vi "诊断标定3 - 副本.vi"(8 "CAN端口":u16(ring), 9 "设备索引号":u16(ring), 10 "CAN卡类型":u32(ring)=21) -> ()   [LabVIEW 2013] (continued)
                n2268 = local read "设备索引号"() -> (w2798:u16)
                n2269 = local read "CAN卡类型"() -> (w2799:u32)
                n2270 = local read "CAN端口"() -> (w2797:u16)
                n2271 = Boolean To (0,1)(Boolean=w2794) -> (0, 1=w2791:i16)
                n2272 = Quotient & Remainder(x=w2788, y=w2789) -> (x-y*floor(x/y)=w2785:dbl)  [unwired: 1 out]
                n2273 = Build Array(i16 1 ("元素"), w2791, w2785, w2784, w2783, w2782, 0.0 ("元素")) -> (w2795:dbl[])
                n2274 = call "多帧发送机制(EV05).vi"("can卡类型"=w2799, "设备索引号"=w2798, "CAN端口"=w2797, "命令"=w2793, "板号"=u8 0, "命令序号"=w2781, "输入数据"=w2795) -> ()  [unwired: 1 in, 12 out]
              }
              frame True {
                w2809 = 256.0 ("y")
                w2801 = u32 1 ("命令序号")
                w2813 = u8 192 ("命令")
                n2275 = local read "动作保持时间"() -> (w2810:dbl)
                n2276 = Quotient & Remainder(x=w2810, y=w2809) -> (x-y*floor(x/y)=w2802:dbl, floor(x/y)=w2806:dbl)
                n2277 = Quotient & Remainder(x=w2806, y=w2809) -> (x-y*floor(x/y)=w2803:dbl, floor(x/y)=w2807:dbl)
                n2278 = Quotient & Remainder(x=w2807, y=w2809) -> (x-y*floor(x/y)=w2804:dbl, floor(x/y)=w2808:dbl)
                n2279 = local read "设备索引号"() -> (w2818:u16)
                n2280 = local read "CAN卡类型"() -> (w2819:u32)
                n2281 = local read "CAN端口"() -> (w2817:u16)
                n2282 = Boolean To (0,1)(Boolean=w2814) -> (0, 1=w2811:i16)
                n2283 = Quotient & Remainder(x=w2808, y=w2809) -> (x-y*floor(x/y)=w2805:dbl)  [unwired: 1 out]
                n2284 = Build Array(i16 1 ("元素"), w2811, w2805, w2804, w2803, w2802, 0.0 ("元素")) -> (w2815:dbl[])
                n2285 = call "多帧发送机制(EV05).vi"("can卡类型"=w2819, "设备索引号"=w2818, "CAN端口"=w2817, "命令"=w2813, "板号"=u8 0, "命令序号"=w2801, "输入数据"=w2815) -> ()  [unwired: 1 in, 12 out]
              }
            }
            n2286 = local write "命令序号"(w2773) -> ()
            n2287 = local write "命令"(w2778) -> ()
            n2288 = local write "控制1"(TRUE ("控制1")) -> ()
            n2289 = local write "写?"(FALSE ("写?")) -> ()
            n2290 = global write "EV05全局变量1.vi" "流控帧"(FALSE ("流控帧")) -> ()
            n2291 = local write "消除"(TRUE ("消除")) -> ()
            n2292 = global write "EV05全局变量1.vi" "流控帧 2"(TRUE ("流控帧 2")) -> ()
          }
          frame #2 {
            n2293 = flat-sequence {
              tunnel: [w2821] -> w2820
              tunnel: w2820 -> [w2828]
              frame #0 {
                n2294 = while {
                  tunnel: [w2822] -> w2821
                  i -> [w2826]
                  stop <- w2823 stop-if-true
                  n2295 = local read "继电器超时处理"() -> (w2822:bool)
                  n2296 = Greater Or Equal?(x=w2826, y=20) -> (x >= y?=w2824:bool)
                  n2297 = Wait Until Next ms Multiple(millisecond multiple=u32 100 ("毫秒倍数")) -> ()  [unwired: 1 out]
                  n2298 = Or(x=w2822, y=w2824) -> (x .or. y?=w2823:bool)
                }
              }
              frame #1 {
                n2299 = case shown="假" w2828 {
                  frame False {
                    n2300 = local read "正级继电器"() -> (w2830:bool)
                    n2301 = Not(x=w2830) -> (.not. x?=w2829:bool)
                    n2302 = local write "正级继电器"(w2829) -> ()
                    n2303 = One Button Dialog(message="继电器处理超时" ("消息"), button name ("OK")="是" ("按钮名称（“确定”）")) -> ()  [unwired: 1 out]
                  }
                  frame True {
                  }
                }
              }
            }
          }
        }
      }
      event "负级继电器": Value Change {
        n2304 = event-data() -> ("NewVal"=w2833:bool)  [unwired: 6 out]
        n2305 = stacked-sequence {
          tunnel: w2833 -> [_ w2846 _]
          frame #0 {
            w2836 = FALSE ("继电器超时处理")
            n2306 = local write "继电器超时处理"(w2836) -> ()
            n2307 = local write "正级继电器 2"(w2836) -> ()
            n2308 = local write "主从选择"(enum32{"主板", "从板"}."主板" ("主从选择")) -> ()
          }
          frame #1 {
            n2309 = case shown="假" w2846 {
              selector: w2846 -> [w2860 w2880]
              tunnel: [w2859 w2879] -> w2845
              tunnel: [w2848 w2868] -> w2840
              frame False {
                w2856 = 256.0 ("y")
                w2848 = u32 1 ("命令序号")
                w2859 = u8 192 ("命令")
                n2310 = local read "动作保持时间"() -> (w2857:dbl)
                n2311 = Quotient & Remainder(x=w2857, y=w2856) -> (x-y*floor(x/y)=w2849:dbl, floor(x/y)=w2853:dbl)
                n2312 = Quotient & Remainder(x=w2853, y=w2856) -> (x-y*floor(x/y)=w2850:dbl, floor(x/y)=w2854:dbl)
                n2313 = Quotient & Remainder(x=w2854, y=w2856) -> (x-y*floor(x/y)=w2851:dbl, floor(x/y)=w2855:dbl)
                n2314 = Quotient & Remainder(x=w2855, y=w2856) -> (x-y*floor(x/y)=w2852:dbl)  [unwired: 1 out]
                n2315 = Boolean To (0,1)(Boolean=w2860) -> (0, 1=w2858:i16)
                n2316 = local read "设备索引号"() -> (w2865:u16)
                n2317 = local read "CAN卡类型"() -> (w2866:u32)
                n2318 = local read "CAN端口"() -> (w2864:u16)
                n2319 = Build Array(i16 2 ("元素"), w2858, w2852, w2851, w2850, w2849, 0.0 ("元素")) -> (w2862:dbl[])
                n2320 = call "多帧发送机制(EV05).vi"("can卡类型"=w2866, "设备索引号"=w2865, "CAN端口"=w2864, "命令"=w2859, "板号"=u8 0, "命令序号"=w2848, "输入数据"=w2862) -> ()  [unwired: 1 in, 12 out]
              }
              frame True {
                w2876 = 256.0 ("y")
                w2868 = u32 1 ("命令序号")
                w2879 = u8 192 ("命令")
                n2321 = local read "动作保持时间"() -> (w2877:dbl)
                n2322 = Quotient & Remainder(x=w2877, y=w2876) -> (x-y*floor(x/y)=w2869:dbl, floor(x/y)=w2873:dbl)
                n2323 = Quotient & Remainder(x=w2873, y=w2876) -> (x-y*floor(x/y)=w2870:dbl, floor(x/y)=w2874:dbl)
                n2324 = Quotient & Remainder(x=w2874, y=w2876) -> (x-y*floor(x/y)=w2871:dbl, floor(x/y)=w2875:dbl)
                n2325 = Quotient & Remainder(x=w2875, y=w2876) -> (x-y*floor(x/y)=w2872:dbl)  [unwired: 1 out]
                n2326 = Boolean To (0,1)(Boolean=w2880) -> (0, 1=w2878:i16)
                n2327 = local read "设备索引号"() -> (w2885:u16)
                n2328 = local read "CAN卡类型"() -> (w2886:u32)
                n2329 = local read "CAN端口"() -> (w2884:u16)
                n2330 = Build Array(i16 2 ("元素"), w2878, w2872, w2871, w2870, w2869, 0.0 ("元素")) -> (w2882:dbl[])
                n2331 = call "多帧发送机制(EV05).vi"("can卡类型"=w2886, "设备索引号"=w2885, "CAN端口"=w2884, "命令"=w2879, "板号"=u8 0, "命令序号"=w2868, "输入数据"=w2882) -> ()  [unwired: 1 in, 12 out]
              }
            }
            n2332 = local write "命令"(w2845) -> ()
            n2333 = local write "命令序号"(w2840) -> ()
            n2334 = local write "清BUFF"(FALSE ("清BUFF")) -> ()
            n2335 = global write "EV05全局变量1.vi" "流控帧"(FALSE ("流控帧")) -> ()
            n2336 = local write "控制1"(TRUE ("控制1")) -> ()
            n2337 = global write "EV05全局变量1.vi" "流控帧 2"(TRUE ("流控帧 2")) -> ()
            n2338 = local write "写?"(FALSE ("写?")) -> ()
            n2339 = local write "消除"(TRUE ("消除")) -> ()
          }
          frame #2 {
            n2340 = flat-sequence {
              tunnel: [w2888] -> w2887
              tunnel: w2887 -> [w2895]
              frame #0 {
                n2341 = while {
                  tunnel: [w2889] -> w2888
                  i -> [w2893]
                  stop <- w2890 stop-if-true
                  n2342 = local read "继电器超时处理"() -> (w2889:bool)
                  n2343 = Greater Or Equal?(x=w2893, y=20) -> (x >= y?=w2891:bool)
                  n2344 = Wait Until Next ms Multiple(millisecond multiple=u32 100 ("毫秒倍数")) -> ()  [unwired: 1 out]
                  n2345 = Or(x=w2889, y=w2891) -> (x .or. y?=w2890:bool)
                }
              }
              frame #1 {
                n2346 = case shown="假" w2895 {
                  frame False {
                    n2347 = local read "负级继电器"() -> (w2896:bool)
                    n2348 = Not(x=w2896) -> (.not. x?=w2897:bool)
                    n2349 = local write "负级继电器"(w2897) -> ()
                    n2350 = One Button Dialog(message="继电器处理超时" ("消息"), button name ("OK")="是" ("按钮名称（“确定”）")) -> ()  [unwired: 1 out]
                  }
                  frame True {
                  }
                }
              }
            }
          }
        }
      }
      event "预充电继电器": Value Change {
        n2351 = event-data() -> ("NewVal"=w2900:bool)  [unwired: 6 out]
        n2352 = stacked-sequence {
          tunnel: w2900 -> [_ w2913 _]
          frame #0 {
            w2904 = FALSE ("继电器超时处理")
            n2353 = local write "继电器超时处理"(w2904) -> ()
            n2354 = local write "正级继电器 3"(w2904) -> ()
            n2355 = global write "EV05全局变量1.vi" "流控帧"(FALSE ("流控帧")) -> ()
            n2356 = local write "主从选择"(enum32{"主板", "从板"}."主板" ("主从选择")) -> ()
          }
          frame #1 {
            n2357 = case shown="假" w2913 {
              selector: w2913 -> [w2927 w2947]
              tunnel: [w2926 w2946] -> w2912
              tunnel: [w2915 w2935] -> w2907
              frame False {
                w2923 = 256.0 ("y")
                w2915 = u32 1 ("命令序号")
                w2926 = u8 192 ("命令")
                n2358 = local read "动作保持时间"() -> (w2924:dbl)
                n2359 = Quotient & Remainder(x=w2924, y=w2923) -> (x-y*floor(x/y)=w2916:dbl, floor(x/y)=w2920:dbl)
                n2360 = Quotient & Remainder(x=w2920, y=w2923) -> (x-y*floor(x/y)=w2917:dbl, floor(x/y)=w2921:dbl)
                n2361 = Quotient & Remainder(x=w2921, y=w2923) -> (x-y*floor(x/y)=w2918:dbl, floor(x/y)=w2922:dbl)
                n2362 = Quotient & Remainder(x=w2922, y=w2923) -> (x-y*floor(x/y)=w2919:dbl)  [unwired: 1 out]
                n2363 = Boolean To (0,1)(Boolean=w2927) -> (0, 1=w2925:i16)
                n2364 = local read "设备索引号"() -> (w2932:u16)
                n2365 = local read "CAN卡类型"() -> (w2933:u32)
                n2366 = local read "CAN端口"() -> (w2931:u16)
                n2367 = Build Array(i16 3 ("元素"), w2925, w2919, w2918, w2917, w2916, 0.0 ("元素")) -> (w2929:dbl[])
                n2368 = call "多帧发送机制(EV05).vi"("can卡类型"=w2933, "设备索引号"=w2932, "CAN端口"=w2931, "命令"=w2926, "板号"=u8 0, "命令序号"=w2915, "输入数据"=w2929) -> ()  [unwired: 1 in, 12 out]
              }
              frame True {
                w2943 = 256.0 ("y")
                w2935 = u32 1 ("命令序号")
                w2946 = u8 192 ("命令")
                n2369 = local read "动作保持时间"() -> (w2944:dbl)
                n2370 = Quotient & Remainder(x=w2944, y=w2943) -> (x-y*floor(x/y)=w2936:dbl, floor(x/y)=w2940:dbl)
                n2371 = Quotient & Remainder(x=w2940, y=w2943) -> (x-y*floor(x/y)=w2937:dbl, floor(x/y)=w2941:dbl)
                n2372 = Quotient & Remainder(x=w2941, y=w2943) -> (x-y*floor(x/y)=w2938:dbl, floor(x/y)=w2942:dbl)
                n2373 = Quotient & Remainder(x=w2942, y=w2943) -> (x-y*floor(x/y)=w2939:dbl)  [unwired: 1 out]
                n2374 = Boolean To (0,1)(Boolean=w2947) -> (0, 1=w2945:i16)
                n2375 = local read "设备索引号"() -> (w2952:u16)
                n2376 = local read "CAN卡类型"() -> (w2953:u32)
                n2377 = local read "CAN端口"() -> (w2951:u16)
                n2378 = Build Array(i16 3 ("元素"), w2945, w2939, w2938, w2937, w2936, 0.0 ("元素")) -> (w2949:dbl[])
                n2379 = call "多帧发送机制(EV05).vi"("can卡类型"=w2953, "设备索引号"=w2952, "CAN端口"=w2951, "命令"=w2946, "板号"=u8 0, "命令序号"=w2935, "输入数据"=w2949) -> ()  [unwired: 1 in, 12 out]
              }
            }
            n2380 = local write "命令序号"(w2907) -> ()
            n2381 = local write "清BUFF"(FALSE ("清BUFF")) -> ()
            n2382 = local write "控制1"(TRUE ("控制1")) -> ()
            n2383 = global write "EV05全局变量1.vi" "流控帧 2"(TRUE ("流控帧 2")) -> ()
            n2384 = local write "消除"(TRUE ("消除")) -> ()
            n2385 = local write "命令"(w2912) -> ()
            n2386 = local write "写?"(FALSE ("写?")) -> ()
          }
          frame #2 {
            n2387 = flat-sequence {
              tunnel: [w2955] -> w2954
              tunnel: w2954 -> [w2962]
              frame #0 {
                n2388 = while {
                  tunnel: [w2956] -> w2955
                  i -> [w2960]
                  stop <- w2957 stop-if-true
                  n2389 = local read "继电器超时处理"() -> (w2956:bool)
                  n2390 = Greater Or Equal?(x=w2960, y=20) -> (x >= y?=w2958:bool)
                  n2391 = Wait Until Next ms Multiple(millisecond multiple=u32 100 ("毫秒倍数")) -> ()  [unwired: 1 out]
                  n2392 = Or(x=w2956, y=w2958) -> (x .or. y?=w2957:bool)
                }
              }
              frame #1 {
                n2393 = case shown="假" w2962 {
                  frame False {
                    n2394 = local read "预充电继电器"() -> (w2963:bool)
                    n2395 = Not(x=w2963) -> (.not. x?=w2964:bool)
                    n2396 = local write "预充电继电器"(w2964) -> ()
                    n2397 = One Button Dialog(message="继电器处理超时" ("消息"), button name ("OK")="是" ("按钮名称（“确定”）")) -> ()  [unwired: 1 out]
                  }
                  frame True {
                  }
                }
              }
            }
          }
        }
      }
      event "加热继电器": Value Change {
        n2398 = event-data() -> ("NewVal"=w2967:bool)  [unwired: 6 out]
        n2399 = stacked-sequence {
          tunnel: w2967 -> [_ w2980 _]
          frame #0 {
            w2971 = FALSE ("继电器超时处理")
            n2400 = local write "继电器超时处理"(w2971) -> ()
            n2401 = local write "正级继电器 5"(w2971) -> ()
            n2402 = global write "EV05全局变量1.vi" "流控帧"(FALSE ("流控帧")) -> ()
            n2403 = local write "主从选择"(enum32{"主板", "从板"}."主板" ("主从选择")) -> ()
          }
          frame #1 {
            n2404 = case shown="假" w2980 {
              selector: w2980 -> [w2994 w3014]
              tunnel: [w2993 w3013] -> w2979
              tunnel: [w2982 w3002] -> w2974
              frame False {
                w2990 = 256.0 ("y")
                w2982 = u32 1 ("命令序号")
                w2993 = u8 192 ("命令")
                n2405 = local read "动作保持时间"() -> (w2991:dbl)
                n2406 = Quotient & Remainder(x=w2991, y=w2990) -> (x-y*floor(x/y)=w2983:dbl, floor(x/y)=w2987:dbl)
                n2407 = Quotient & Remainder(x=w2987, y=w2990) -> (x-y*floor(x/y)=w2984:dbl, floor(x/y)=w2988:dbl)
                n2408 = Quotient & Remainder(x=w2988, y=w2990) -> (x-y*floor(x/y)=w2985:dbl, floor(x/y)=w2989:dbl)
                n2409 = Quotient & Remainder(x=w2989, y=w2990) -> (x-y*floor(x/y)=w2986:dbl)  [unwired: 1 out]
                n2410 = Boolean To (0,1)(Boolean=w2994) -> (0, 1=w2992:i16)
                n2411 = local read "设备索引号"() -> (w2999:u16)
                n2412 = local read "CAN卡类型"() -> (w3000:u32)
                n2413 = local read "CAN端口"() -> (w2998:u16)
                n2414 = Build Array(i16 4 ("元素"), w2992, w2986, w2985, w2984, w2983, 0.0 ("元素")) -> (w2996:dbl[])
                n2415 = call "多帧发送机制(EV05).vi"("can卡类型"=w3000, "设备索引号"=w2999, "CAN端口"=w2998, "命令"=w2993, "板号"=u8 0, "命令序号"=w2982, "输入数据"=w2996) -> ()  [unwired: 1 in, 12 out]
              }
              frame True {
                w3010 = 256.0 ("y")
                w3002 = u32 1 ("命令序号")
                w3013 = u8 192 ("命令")
                n2416 = local read "动作保持时间"() -> (w3011:dbl)
                n2417 = Quotient & Remainder(x=w3011, y=w3010) -> (x-y*floor(x/y)=w3003:dbl, floor(x/y)=w3007:dbl)
                n2418 = Quotient & Remainder(x=w3007, y=w3010) -> (x-y*floor(x/y)=w3004:dbl, floor(x/y)=w3008:dbl)
                n2419 = Quotient & Remainder(x=w3008, y=w3010) -> (x-y*floor(x/y)=w3005:dbl, floor(x/y)=w3009:dbl)
                n2420 = Quotient & Remainder(x=w3009, y=w3010) -> (x-y*floor(x/y)=w3006:dbl)  [unwired: 1 out]
                n2421 = Boolean To (0,1)(Boolean=w3014) -> (0, 1=w3012:i16)
                n2422 = local read "设备索引号"() -> (w3019:u16)
                n2423 = local read "CAN卡类型"() -> (w3020:u32)
                n2424 = local read "CAN端口"() -> (w3018:u16)
                n2425 = Build Array(i16 4 ("元素"), w3012, w3006, w3005, w3004, w3003, 0.0 ("元素")) -> (w3016:dbl[])
                n2426 = call "多帧发送机制(EV05).vi"("can卡类型"=w3020, "设备索引号"=w3019, "CAN端口"=w3018, "命令"=w3013, "板号"=u8 0, "命令序号"=w3002, "输入数据"=w3016) -> ()  [unwired: 1 in, 12 out]
              }
            }
            n2427 = local write "命令序号"(w2974) -> ()
            n2428 = local write "清BUFF"(FALSE ("清BUFF")) -> ()
            n2429 = local write "命令"(w2979) -> ()
            n2430 = local write "控制1"(TRUE ("控制1")) -> ()
            n2431 = local write "写?"(FALSE ("写?")) -> ()
            n2432 = global write "EV05全局变量1.vi" "流控帧 2"(TRUE ("流控帧 2")) -> ()
            n2433 = local write "消除"(TRUE ("消除")) -> ()
          }
          frame #2 {
            n2434 = flat-sequence {
              tunnel: [w3022] -> w3021
              tunnel: w3021 -> [w3029]
              frame #0 {
                n2435 = while {
                  tunnel: [w3023] -> w3022
                  i -> [w3027]
                  stop <- w3024 stop-if-true
                  n2436 = local read "继电器超时处理"() -> (w3023:bool)
                  n2437 = Greater Or Equal?(x=w3027, y=20) -> (x >= y?=w3025:bool)
                  n2438 = Wait Until Next ms Multiple(millisecond multiple=u32 100 ("毫秒倍数")) -> ()  [unwired: 1 out]
                  n2439 = Or(x=w3023, y=w3025) -> (x .or. y?=w3024:bool)
                }
              }
              frame #1 {
                n2440 = case shown="假" w3029 {
                  frame False {
                    n2441 = local read "加热继电器"() -> (w3030:bool)
                    n2442 = Not(x=w3030) -> (.not. x?=w3031:bool)
                    n2443 = local write "加热继电器"(w3031) -> ()
                    n2444 = One Button Dialog(message="继电器处理超时" ("消息"), button name ("OK")="是" ("按钮名称（“确定”）")) -> ()  [unwired: 1 out]
                  }
                  frame True {
                  }
                }
              }
            }
          }
        }
      }
      event "充电继电器": Value Change {
        n2445 = event-data() -> ("NewVal"=w3034:bool)  [unwired: 6 out]
        n2446 = stacked-sequence {
          tunnel: w3034 -> [_ w3047 _]
          frame #0 {
            w3038 = FALSE ("继电器超时处理")
            n2447 = local write "主从选择"(enum32{"主板", "从板"}."主板" ("主从选择")) -> ()
            n2448 = global write "EV05全局变量1.vi" "流控帧"(FALSE ("流控帧")) -> ()
            n2449 = local write "继电器超时处理"(w3038) -> ()
            n2450 = local write "正级继电器 4"(w3038) -> ()
          }
          frame #1 {
            n2451 = case shown="假" w3047 {
              selector: w3047 -> [w3061 w3081]
              tunnel: [w3060 w3080] -> w3046
              tunnel: [w3049 w3069] -> w3041
              frame False {
                w3057 = 256.0 ("y")
                w3049 = u32 1 ("命令序号")
                w3060 = u8 192 ("命令")
                n2452 = local read "动作保持时间"() -> (w3058:dbl)
                n2453 = Quotient & Remainder(x=w3058, y=w3057) -> (x-y*floor(x/y)=w3050:dbl, floor(x/y)=w3054:dbl)
                n2454 = Quotient & Remainder(x=w3054, y=w3057) -> (x-y*floor(x/y)=w3051:dbl, floor(x/y)=w3055:dbl)
                n2455 = Quotient & Remainder(x=w3055, y=w3057) -> (x-y*floor(x/y)=w3052:dbl, floor(x/y)=w3056:dbl)
                n2456 = Quotient & Remainder(x=w3056, y=w3057) -> (x-y*floor(x/y)=w3053:dbl)  [unwired: 1 out]
                n2457 = Boolean To (0,1)(Boolean=w3061) -> (0, 1=w3059:i16)
                n2458 = local read "设备索引号"() -> (w3066:u16)
                n2459 = local read "CAN卡类型"() -> (w3067:u32)
                n2460 = local read "CAN端口"() -> (w3065:u16)
                n2461 = Build Array(i16 5 ("元素"), w3059, w3053, w3052, w3051, w3050, 0.0 ("元素")) -> (w3063:dbl[])
                n2462 = call "多帧发送机制(EV05).vi"("can卡类型"=w3067, "设备索引号"=w3066, "CAN端口"=w3065, "命令"=w3060, "板号"=u8 0, "命令序号"=w3049, "输入数据"=w3063) -> ()  [unwired: 1 in, 12 out]
              }
              frame True {
                w3077 = 256.0 ("y")
                w3069 = u32 1 ("命令序号")
                w3080 = u8 192 ("命令")
                n2463 = local read "动作保持时间"() -> (w3078:dbl)
                n2464 = Quotient & Remainder(x=w3078, y=w3077) -> (x-y*floor(x/y)=w3070:dbl, floor(x/y)=w3074:dbl)
                n2465 = Quotient & Remainder(x=w3074, y=w3077) -> (x-y*floor(x/y)=w3071:dbl, floor(x/y)=w3075:dbl)
                n2466 = Quotient & Remainder(x=w3075, y=w3077) -> (x-y*floor(x/y)=w3072:dbl, floor(x/y)=w3076:dbl)
                n2467 = Quotient & Remainder(x=w3076, y=w3077) -> (x-y*floor(x/y)=w3073:dbl)  [unwired: 1 out]
                n2468 = Boolean To (0,1)(Boolean=w3081) -> (0, 1=w3079:i16)
                n2469 = local read "设备索引号"() -> (w3086:u16)
                n2470 = local read "CAN卡类型"() -> (w3087:u32)
                n2471 = local read "CAN端口"() -> (w3085:u16)
                n2472 = Build Array(i16 5 ("元素"), w3079, w3073, w3072, w3071, w3070, 0.0 ("元素")) -> (w3083:dbl[])
                n2473 = call "多帧发送机制(EV05).vi"("can卡类型"=w3087, "设备索引号"=w3086, "CAN端口"=w3085, "命令"=w3080, "板号"=u8 0, "命令序号"=w3069, "输入数据"=w3083) -> ()  [unwired: 1 in, 12 out]
              }
            }
            n2474 = local write "命令序号"(w3041) -> ()
            n2475 = local write "命令"(w3046) -> ()
            n2476 = local write "清BUFF"(FALSE ("清BUFF")) -> ()
            n2477 = local write "控制1"(TRUE ("控制1")) -> ()
            n2478 = global write "EV05全局变量1.vi" "流控帧 2"(TRUE ("流控帧 2")) -> ()
            n2479 = local write "写?"(FALSE ("写?")) -> ()
            n2480 = local write "消除"(TRUE ("消除")) -> ()
          }
          frame #2 {
            n2481 = flat-sequence {
              tunnel: [w3089] -> w3088
              tunnel: w3088 -> [w3096]
              frame #0 {
                n2482 = while {
                  tunnel: [w3090] -> w3089
                  i -> [w3094]
                  stop <- w3091 stop-if-true
                  n2483 = local read "继电器超时处理"() -> (w3090:bool)
                  n2484 = Greater Or Equal?(x=w3094, y=20) -> (x >= y?=w3092:bool)
                  n2485 = Wait Until Next ms Multiple(millisecond multiple=u32 100 ("毫秒倍数")) -> ()  [unwired: 1 out]
                  n2486 = Or(x=w3090, y=w3092) -> (x .or. y?=w3091:bool)
                }
              }
              frame #1 {
                n2487 = case shown="假" w3096 {
                  frame False {
                    n2488 = local read "充电继电器"() -> (w3097:bool)
                    n2489 = Not(x=w3097) -> (.not. x?=w3098:bool)
                    n2490 = local write "充电继电器"(w3098) -> ()
                    n2491 = One Button Dialog(message="继电器处理超时" ("消息"), button name ("OK")="是" ("按钮名称（“确定”）")) -> ()  [unwired: 1 out]
                  }
                  frame True {
                  }
                }
              }
            }
          }
        }
      }
      event "风机继电器": Value Change {
        n2492 = event-data() -> ("NewVal"=w3101:bool)  [unwired: 6 out]
        n2493 = stacked-sequence {
          tunnel: w3101 -> [_ w3114 _]
          frame #0 {
            w3105 = FALSE ("继电器超时处理")
            n2494 = local write "继电器超时处理"(w3105) -> ()
            n2495 = local write "正级继电器 6"(w3105) -> ()
            n2496 = global write "EV05全局变量1.vi" "流控帧"(FALSE ("流控帧")) -> ()
            n2497 = local write "主从选择"(enum32{"主板", "从板"}."主板" ("主从选择")) -> ()
          }
          frame #1 {
            n2498 = case shown="真" w3114 {
              selector: w3114 -> [w3128 w3148]
              tunnel: [w3127 w3147] -> w3113
              tunnel: [w3116 w3136] -> w3108
              frame True {
                w3124 = 256.0 ("y")
                w3116 = u32 1 ("命令序号")
                w3127 = u8 192 ("命令")
                n2499 = local read "动作保持时间"() -> (w3125:dbl)
                n2500 = Quotient & Remainder(x=w3125, y=w3124) -> (x-y*floor(x/y)=w3117:dbl, floor(x/y)=w3121:dbl)
                n2501 = Quotient & Remainder(x=w3121, y=w3124) -> (x-y*floor(x/y)=w3118:dbl, floor(x/y)=w3122:dbl)
                n2502 = Quotient & Remainder(x=w3122, y=w3124) -> (x-y*floor(x/y)=w3119:dbl, floor(x/y)=w3123:dbl)
                n2503 = Boolean To (0,1)(Boolean=w3128) -> (0, 1=w3126:i16)
                n2504 = local read "设备索引号"() -> (w3133:u16)
                n2505 = local read "CAN卡类型"() -> (w3134:u32)
                n2506 = Quotient & Remainder(x=w3123, y=w3124) -> (x-y*floor(x/y)=w3120:dbl)  [unwired: 1 out]
                n2507 = local read "CAN端口"() -> (w3132:u16)
                n2508 = Build Array(i16 6 ("元素"), w3126, w3120, w3119, w3118, w3117, 0.0 ("元素")) -> (w3130:dbl[])
                n2509 = call "多帧发送机制(EV05).vi"("can卡类型"=w3134, "设备索引号"=w3133, "CAN端口"=w3132, "命令"=w3127, "板号"=u8 0, "命令序号"=w3116, "输入数据"=w3130) -> ()  [unwired: 1 in, 12 out]
              }
              frame False {
                w3144 = 256.0 ("y")
                w3136 = u32 1 ("命令序号")
                w3147 = u8 192 ("命令")
                n2510 = local read "动作保持时间"() -> (w3145:dbl)
                n2511 = Quotient & Remainder(x=w3145, y=w3144) -> (x-y*floor(x/y)=w3137:dbl, floor(x/y)=w3141:dbl)
                n2512 = Quotient & Remainder(x=w3141, y=w3144) -> (x-y*floor(x/y)=w3138:dbl, floor(x/y)=w3142:dbl)
                n2513 = Quotient & Remainder(x=w3142, y=w3144) -> (x-y*floor(x/y)=w3139:dbl, floor(x/y)=w3143:dbl)
                n2514 = Boolean To (0,1)(Boolean=w3148) -> (0, 1=w3146:i16)
                n2515 = local read "设备索引号"() -> (w3153:u16)
                n2516 = local read "CAN卡类型"() -> (w3154:u32)
                n2517 = Quotient & Remainder(x=w3143, y=w3144) -> (x-y*floor(x/y)=w3140:dbl)  [unwired: 1 out]
                n2518 = local read "CAN端口"() -> (w3152:u16)
                n2519 = Build Array(i16 6 ("元素"), w3146, w3140, w3139, w3138, w3137, 0.0 ("元素")) -> (w3150:dbl[])
                n2520 = call "多帧发送机制(EV05).vi"("can卡类型"=w3154, "设备索引号"=w3153, "CAN端口"=w3152, "命令"=w3147, "板号"=u8 0, "命令序号"=w3136, "输入数据"=w3150) -> ()  [unwired: 1 in, 12 out]
              }
            }
            n2521 = local write "命令序号"(w3108) -> ()
            n2522 = local write "命令"(w3113) -> ()
            n2523 = local write "清BUFF"(FALSE ("清BUFF")) -> ()
            n2524 = local write "控制1"(TRUE ("控制1")) -> ()
            n2525 = global write "EV05全局变量1.vi" "流控帧 2"(TRUE ("流控帧 2")) -> ()
            n2526 = local write "写?"(FALSE ("写?")) -> ()
            n2527 = local write "消除"(TRUE ("消除")) -> ()
          }
          frame #2 {
            n2528 = flat-sequence {
              tunnel: [w3156] -> w3155
              tunnel: w3155 -> [w3163]
              frame #0 {
                n2529 = while {
                  tunnel: [w3157] -> w3156
                  i -> [w3161]
                  stop <- w3158 stop-if-true
                  n2530 = local read "继电器超时处理"() -> (w3157:bool)
                  n2531 = Greater Or Equal?(x=w3161, y=20) -> (x >= y?=w3159:bool)
                  n2532 = Wait Until Next ms Multiple(millisecond multiple=u32 100 ("毫秒倍数")) -> ()  [unwired: 1 out]
                  n2533 = Or(x=w3157, y=w3159) -> (x .or. y?=w3158:bool)
                }
              }
              frame #1 {
                n2534 = case shown="假" w3163 {
                  frame False {
                    n2535 = local read "风机继电器"() -> (w3164:bool)
                    n2536 = Not(x=w3164) -> (.not. x?=w3165:bool)
                    n2537 = local write "风机继电器"(w3165) -> ()
                    n2538 = One Button Dialog(message="继电器处理超时" ("消息"), button name ("OK")="是" ("按钮名称（“确定”）")) -> ()  [unwired: 1 out]
                  }
                  frame True {
                  }
                }
              }
            }
          }
        }
      }
      event "加热继电器(从)": Value Change {
        n2539 = event-data() -> ("NewVal"=w3168:bool)  [unwired: 6 out]
        n2540 = stacked-sequence {
          tunnel: w3168 -> [_ w3182 _]
          frame #0 {
            w3172 = FALSE ("继电器超时处理")
            n2541 = local write "正级继电器 7"(w3172) -> ()
            n2542 = local write "继电器超时处理"(w3172) -> ()
            n2543 = global write "EV05全局变量1.vi" "流控帧"(FALSE ("流控帧")) -> ()
            n2544 = local write "主从选择"(enum32{"主板", "从板"}."从板" ("主从选择")) -> ()
          }
          frame #1 {
            n2545 = case shown="真" w3182 {
              selector: w3182 -> [w3197 w3217]
              tunnel: [w3196 w3216] -> w3181
              tunnel: [w3195 w3215] -> w3175
              tunnel: [w3184 w3204] -> w3176
              frame True {
                w3192 = 256.0 ("y")
                w3184 = u32 1 ("命令序号")
                w3196 = u8 192 ("命令")
                n2546 = local read "动作保持时间"() -> (w3193:dbl)
                n2547 = Quotient & Remainder(x=w3193, y=w3192) -> (x-y*floor(x/y)=w3185:dbl, floor(x/y)=w3189:dbl)
                n2548 = Quotient & Remainder(x=w3189, y=w3192) -> (x-y*floor(x/y)=w3186:dbl, floor(x/y)=w3190:dbl)
                n2549 = Quotient & Remainder(x=w3190, y=w3192) -> (x-y*floor(x/y)=w3187:dbl, floor(x/y)=w3191:dbl)
                n2550 = Quotient & Remainder(x=w3191, y=w3192) -> (x-y*floor(x/y)=w3188:dbl)  [unwired: 1 out]
                n2551 = Boolean To (0,1)(Boolean=w3197) -> (0, 1=w3194:i16)
                n2552 = local read "设备索引号"() -> (w3201:u16)
                n2553 = local read "CAN卡类型"() -> (w3202:u32)
                n2554 = local read "从板板号"() -> (w3195:u8)
                n2555 = local read "CAN端口"() -> (w3200:u16)
                n2556 = Build Array(i16 7 ("元素"), w3194, w3188, w3187, w3186, w3185, 0.0 ("元素")) -> (w3199:dbl[])
                n2557 = call "多帧发送机制(EV05).vi"("can卡类型"=w3202, "设备索引号"=w3201, "CAN端口"=w3200, "命令"=w3196, "板号"=w3195, "命令序号"=w3184, "输入数据"=w3199) -> ()  [unwired: 1 in, 12 out]
              }
              frame False {
                w3212 = 256.0 ("y")
                w3204 = u32 1 ("命令序号")
                w3216 = u8 192 ("命令")
                n2558 = local read "动作保持时间"() -> (w3213:dbl)
                n2559 = Quotient & Remainder(x=w3213, y=w3212) -> (x-y*floor(x/y)=w3205:dbl, floor(x/y)=w3209:dbl)
                n2560 = Quotient & Remainder(x=w3209, y=w3212) -> (x-y*floor(x/y)=w3206:dbl, floor(x/y)=w3210:dbl)
                n2561 = Quotient & Remainder(x=w3210, y=w3212) -> (x-y*floor(x/y)=w3207:dbl, floor(x/y)=w3211:dbl)
                n2562 = Quotient & Remainder(x=w3211, y=w3212) -> (x-y*floor(x/y)=w3208:dbl)  [unwired: 1 out]
                n2563 = Boolean To (0,1)(Boolean=w3217) -> (0, 1=w3214:i16)
                n2564 = local read "设备索引号"() -> (w3221:u16)
                n2565 = local read "CAN卡类型"() -> (w3222:u32)
                n2566 = local read "从板板号"() -> (w3215:u8)
                n2567 = local read "CAN端口"() -> (w3220:u16)
                n2568 = Build Array(i16 7 ("元素"), w3214, w3208, w3207, w3206, w3205, 0.0 ("元素")) -> (w3219:dbl[])
                n2569 = call "多帧发送机制(EV05).vi"("can卡类型"=w3222, "设备索引号"=w3221, "CAN端口"=w3220, "命令"=w3216, "板号"=w3215, "命令序号"=w3204, "输入数据"=w3219) -> ()  [unwired: 1 in, 12 out]
              }
            }
            n2570 = local write "从板板号"(w3175) -> ()
            n2571 = local write "命令序号"(w3176) -> ()
            n2572 = local write "命令"(w3181) -> ()
            n2573 = local write "清BUFF"(FALSE ("清BUFF")) -> ()
            n2574 = local write "写?"(FALSE ("写?")) -> ()
            n2575 = local write "控制1"(TRUE ("控制1")) -> ()
            n2576 = global write "EV05全局变量1.vi" "流控帧 2"(TRUE ("流控帧 2")) -> ()
            n2577 = local write "消除"(TRUE ("消除")) -> ()
          }
          frame #2 {
            n2578 = flat-sequence {
              tunnel: [w3224] -> w3223
              tunnel: w3223 -> [w3231]
              frame #0 {
                n2579 = while {
                  tunnel: [w3225] -> w3224
                  i -> [w3229]
                  stop <- w3226 stop-if-true
                  n2580 = local read "继电器超时处理"() -> (w3225:bool)
                  n2581 = Greater Or Equal?(x=w3229, y=20) -> (x >= y?=w3227:bool)
                  n2582 = Wait Until Next ms Multiple(millisecond multiple=u32 100 ("毫秒倍数")) -> ()  [unwired: 1 out]
                  n2583 = Or(x=w3225, y=w3227) -> (x .or. y?=w3226:bool)
                }
              }
              frame #1 {
                n2584 = case shown="假" w3231 {
                  frame False {
                    n2585 = local read "加热继电器(从)"() -> (w3233:bool)
                    n2586 = Not(x=w3233) -> (.not. x?=w3232:bool)
                    n2587 = local write "加热继电器(从)"(w3232) -> ()
                    n2588 = One Button Dialog(message="继电器处理超时" ("消息"), button name ("OK")="是" ("按钮名称（“确定”）")) -> ()  [unwired: 1 out]
                  }
                  frame True {
                  }
                }
              }
            }
          }
        }
      }
      event "风机继电器(从)": Value Change {
        n2589 = event-data() -> ("NewVal"=w3236:bool)  [unwired: 6 out]
        n2590 = stacked-sequence {
          tunnel: w3236 -> [_ w3250 _]
          frame #0 {
            w3240 = FALSE ("继电器超时处理")
            n2591 = local write "继电器超时处理"(w3240) -> ()
            n2592 = local write "正级继电器 8"(w3240) -> ()
            n2593 = global write "EV05全局变量1.vi" "流控帧"(FALSE ("流控帧")) -> ()
            n2594 = local write "主从选择"(enum32{"主板", "从板"}."从板" ("主从选择")) -> ()
          }
          frame #1 {
            n2595 = case shown="假" w3250 {
              selector: w3250 -> [w3265 w3285]
              tunnel: [w3264 w3284] -> w3249
              tunnel: [w3263 w3283] -> w3243
              tunnel: [w3252 w3272] -> w3244
              frame False {
                w3260 = 256.0 ("y")
                w3252 = u32 1 ("命令序号")
                w3264 = u8 192 ("命令")
                n2596 = local read "动作保持时间"() -> (w3261:dbl)
                n2597 = Quotient & Remainder(x=w3261, y=w3260) -> (x-y*floor(x/y)=w3253:dbl, floor(x/y)=w3257:dbl)
                n2598 = Quotient & Remainder(x=w3257, y=w3260) -> (x-y*floor(x/y)=w3254:dbl, floor(x/y)=w3258:dbl)
                n2599 = Quotient & Remainder(x=w3258, y=w3260) -> (x-y*floor(x/y)=w3255:dbl, floor(x/y)=w3259:dbl)
                n2600 = Quotient & Remainder(x=w3259, y=w3260) -> (x-y*floor(x/y)=w3256:dbl)  [unwired: 1 out]
                n2601 = local read "设备索引号"() -> (w3269:u16)
                n2602 = local read "CAN卡类型"() -> (w3270:u32)
                n2603 = local read "从板板号"() -> (w3263:u8)
                n2604 = Boolean To (0,1)(Boolean=w3265) -> (0, 1=w3262:i16)
                n2605 = local read "CAN端口"() -> (w3268:u16)
                n2606 = Build Array(i16 8 ("元素"), w3262, w3256, w3255, w3254, w3253, 0.0 ("元素")) -> (w3267:dbl[])
                n2607 = call "多帧发送机制(EV05).vi"("can卡类型"=w3270, "设备索引号"=w3269, "CAN端口"=w3268, "命令"=w3264, "板号"=w3263, "命令序号"=w3252, "输入数据"=w3267) -> ()  [unwired: 1 in, 12 out]
              }
              frame True {
                w3280 = 256.0 ("y")
                w3272 = u32 1 ("命令序号")
                w3284 = u8 192 ("命令")
                n2608 = local read "动作保持时间"() -> (w3281:dbl)
                n2609 = Quotient & Remainder(x=w3281, y=w3280) -> (x-y*floor(x/y)=w3273:dbl, floor(x/y)=w3277:dbl)
                n2610 = Quotient & Remainder(x=w3277, y=w3280) -> (x-y*floor(x/y)=w3274:dbl, floor(x/y)=w3278:dbl)
                n2611 = Quotient & Remainder(x=w3278, y=w3280) -> (x-y*floor(x/y)=w3275:dbl, floor(x/y)=w3279:dbl)
                n2612 = Quotient & Remainder(x=w3279, y=w3280) -> (x-y*floor(x/y)=w3276:dbl)  [unwired: 1 out]
                n2613 = local read "设备索引号"() -> (w3289:u16)
                n2614 = local read "CAN卡类型"() -> (w3290:u32)
                n2615 = local read "从板板号"() -> (w3283:u8)
                n2616 = Boolean To (0,1)(Boolean=w3285) -> (0, 1=w3282:i16)
                n2617 = local read "CAN端口"() -> (w3288:u16)
                n2618 = Build Array(i16 8 ("元素"), w3282, w3276, w3275, w3274, w3273, 0.0 ("元素")) -> (w3287:dbl[])
                n2619 = call "多帧发送机制(EV05).vi"("can卡类型"=w3290, "设备索引号"=w3289, "CAN端口"=w3288, "命令"=w3284, "板号"=w3283, "命令序号"=w3272, "输入数据"=w3287) -> ()  [unwired: 1 in, 12 out]
              }
            }
            n2620 = local write "从板板号"(w3243) -> ()
            n2621 = local write "清BUFF"(FALSE ("清BUFF")) -> ()
            n2622 = local write "命令序号"(w3244) -> ()
            n2623 = local write "命令"(w3249) -> ()
            n2624 = local write "控制1"(TRUE ("控制1")) -> ()
            n2625 = local write "写?"(FALSE ("写?")) -> ()
            n2626 = local write "消除"(TRUE ("消除")) -> ()
            n2627 = global write "EV05全局变量1.vi" "流控帧 2"(TRUE ("流控帧 2")) -> ()
          }
          frame #2 {
            n2628 = flat-sequence {
              tunnel: [w3292] -> w3291
              tunnel: w3291 -> [w3299]
              frame #0 {
                n2629 = while {
                  tunnel: [w3293] -> w3292
                  i -> [w3297]
                  stop <- w3294 stop-if-true
                  n2630 = local read "继电器超时处理"() -> (w3293:bool)
                  n2631 = Greater Or Equal?(x=w3297, y=20) -> (x >= y?=w3295:bool)
                  n2632 = Wait Until Next ms Multiple(millisecond multiple=u32 100 ("毫秒倍数")) -> ()  [unwired: 1 out]
                  n2633 = Or(x=w3293, y=w3295) -> (x .or. y?=w3294:bool)
                }
              }
              frame #1 {
                n2634 = case shown="假" w3299 {
                  frame False {
                    n2635 = local read "风机继电器(从)"() -> (w3301:bool)
                    n2636 = Not(x=w3301) -> (.not. x?=w3300:bool)
                    n2637 = local write "风机继电器(从)"(w3300) -> ()
                    n2638 = One Button Dialog(message="继电器处理超时" ("消息"), button name ("OK")="是" ("按钮名称（“确定”）")) -> ()  [unwired: 1 out]
                  }
                  frame True {
                  }
                }
              }
            }
          }
        }
      }
      event "DO1": Value Change {
        n2639 = event-data() -> ("NewVal"=w3304:bool)  [unwired: 6 out]
        n2640 = stacked-sequence {
          tunnel: w3304 -> [_ w3317 _]
          frame #0 {
            w3307 = FALSE ("清BUFF")
            n2641 = local write "继电器超时处理"(FALSE ("继电器超时处理")) -> ()
            n2642 = local write "清BUFF"(w3307) -> ()
            n2643 = local write "正级继电器 9"(w3307) -> ()
            n2644 = local write "主从选择"(enum32{"主板", "从板"}."主板" ("主从选择")) -> ()
          }
          frame #1 {
            n2645 = case shown="真" w3317 {
              selector: w3317 -> [w3332 w3352]
              tunnel: [w3331 w3351] -> w3316
              tunnel: [w3319 w3339] -> w3311
              frame False {
                w3327 = 256.0 ("y")
                w3319 = u32 2 ("命令序号")
                w3331 = u8 192 ("命令")
                n2646 = local read "动作保持时间"() -> (w3328:dbl)
                n2647 = Quotient & Remainder(x=w3328, y=w3327) -> (x-y*floor(x/y)=w3320:dbl, floor(x/y)=w3324:dbl)
                n2648 = Quotient & Remainder(x=w3324, y=w3327) -> (x-y*floor(x/y)=w3321:dbl, floor(x/y)=w3325:dbl)
                n2649 = Quotient & Remainder(x=w3325, y=w3327) -> (x-y*floor(x/y)=w3322:dbl, floor(x/y)=w3326:dbl)
                n2650 = local read "设备索引号"() -> (w3336:u16)
                n2651 = local read "CAN卡类型"() -> (w3337:u32)
                n2652 = local read "CAN端口"() -> (w3335:u16)
                n2653 = Boolean To (0,1)(Boolean=w3332) -> (0, 1=w3329:i16)
                n2654 = Quotient & Remainder(x=w3326, y=w3327) -> (x-y*floor(x/y)=w3323:dbl)  [unwired: 1 out]
                n2655 = Build Array(i16 1 ("元素"), w3329, w3323, w3322, w3321, w3320, 0.0 ("元素")) -> (w3333:dbl[])
                n2656 = call "多帧发送机制(EV05).vi"("can卡类型"=w3337, "设备索引号"=w3336, "CAN端口"=w3335, "命令"=w3331, "板号"=u8 0, "命令序号"=w3319, "输入数据"=w3333) -> ()  [unwired: 1 in, 12 out]
              }
              frame True {
                w3347 = 256.0 ("y")
                w3339 = u32 2 ("命令序号")
                w3351 = u8 192 ("命令")
                n2657 = local read "动作保持时间"() -> (w3348:dbl)
                n2658 = Quotient & Remainder(x=w3348, y=w3347) -> (x-y*floor(x/y)=w3340:dbl, floor(x/y)=w3344:dbl)
                n2659 = Quotient & Remainder(x=w3344, y=w3347) -> (x-y*floor(x/y)=w3341:dbl, floor(x/y)=w3345:dbl)
                n2660 = Quotient & Remainder(x=w3345, y=w3347) -> (x-y*floor(x/y)=w3342:dbl, floor(x/y)=w3346:dbl)
                n2661 = local read "设备索引号"() -> (w3356:u16)
                n2662 = local read "CAN卡类型"() -> (w3357:u32)
                n2663 = local read "CAN端口"() -> (w3355:u16)
                n2664 = Boolean To (0,1)(Boolean=w3352) -> (0, 1=w3349:i16)
                n2665 = Quotient & Remainder(x=w3346, y=w3347) -> (x-y*floor(x/y)=w3343:dbl)  [unwired: 1 out]
                n2666 = Build Array(i16 1 ("元素"), w3349, w3343, w3342, w3341, w3340, 0.0 ("元素")) -> (w3353:dbl[])
                n2667 = call "多帧发送机制(EV05).vi"("can卡类型"=w3357, "设备索引号"=w3356, "CAN端口"=w3355, "命令"=w3351, "板号"=u8 0, "命令序号"=w3339, "输入数据"=w3353) -> ()  [unwired: 1 in, 12 out]
              }
            }
            n2668 = local write "命令序号"(w3311) -> ()
            n2669 = local write "命令"(w3316) -> ()
            n2670 = local write "控制1"(TRUE ("控制1")) -> ()
            n2671 = local write "写?"(FALSE ("写?")) -> ()
            n2672 = local write "消除"(TRUE ("消除")) -> ()
            n2673 = global write "EV05全局变量1.vi" "流控帧 2"(TRUE ("流控帧 2")) -> ()
            n2674 = global write "EV05全局变量1.vi" "流控帧"(FALSE ("流控帧")) -> ()
          }
          frame #2 {
            n2675 = flat-sequence {
              tunnel: [w3359] -> w3358
              tunnel: w3358 -> [w3366]
              frame #0 {
                n2676 = while {
                  tunnel: [w3360] -> w3359
                  i -> [w3364]
                  stop <- w3361 stop-if-true
                  n2677 = local read "继电器超时处理"() -> (w3360:bool)
                  n2678 = Greater Or Equal?(x=w3364, y=20) -> (x >= y?=w3362:bool)
                  n2679 = Wait Until Next ms Multiple(millisecond multiple=u32 100 ("毫秒倍数")) -> ()  [unwired: 1 out]
                  n2680 = Or(x=w3360, y=w3362) -> (x .or. y?=w3361:bool)
                }
              }
              frame #1 {
                n2681 = case shown="假" w3366 {
                  frame False {
                    n2682 = local read "DO1"() -> (w3368:bool)
                    n2683 = Not(x=w3368) -> (.not. x?=w3367:bool)
                    n2684 = local write "DO1"(w3367) -> ()
                    n2685 = One Button Dialog(message="DO控制处理超时" ("消息"), button name ("OK")="是" ("按钮名称（“确定”）")) -> ()  [unwired: 1 out]
                  }
                  frame True {
                  }
                }
              }
            }
          }
        }
      }
      event "DO2": Value Change {
        n2686 = event-data() -> ("NewVal"=w3371:bool)  [unwired: 6 out]
        n2687 = stacked-sequence {
          tunnel: w3371 -> [_ w3384 _]
          frame #0 {
            w3374 = FALSE ("清BUFF")
            n2688 = local write "继电器超时处理"(FALSE ("继电器超时处理")) -> ()
            n2689 = local write "主从选择"(enum32{"主板", "从板"}."主板" ("主从选择")) -> ()
            n2690 = local write "清BUFF"(w3374) -> ()
            n2691 = local write "正级继电器 10"(w3374) -> ()
          }
          frame #1 {
            n2692 = case shown="真" w3384 {
              selector: w3384 -> [w3399 w3419]
              tunnel: [w3398 w3418] -> w3383
              tunnel: [w3386 w3406] -> w3378
              frame False {
                w3394 = 256.0 ("y")
                w3386 = u32 2 ("命令序号")
                w3398 = u8 192 ("命令")
                n2693 = local read "动作保持时间"() -> (w3395:dbl)
                n2694 = Quotient & Remainder(x=w3395, y=w3394) -> (x-y*floor(x/y)=w3387:dbl, floor(x/y)=w3391:dbl)
                n2695 = Quotient & Remainder(x=w3391, y=w3394) -> (x-y*floor(x/y)=w3388:dbl, floor(x/y)=w3392:dbl)
                n2696 = Quotient & Remainder(x=w3392, y=w3394) -> (x-y*floor(x/y)=w3389:dbl, floor(x/y)=w3393:dbl)
                n2697 = local read "设备索引号"() -> (w3403:u16)
                n2698 = local read "CAN卡类型"() -> (w3404:u32)
                n2699 = local read "CAN端口"() -> (w3402:u16)
                n2700 = Boolean To (0,1)(Boolean=w3399) -> (0, 1=w3396:i16)
                n2701 = Quotient & Remainder(x=w3393, y=w3394) -> (x-y*floor(x/y)=w3390:dbl)  [unwired: 1 out]
                n2702 = Build Array(i16 2 ("元素"), w3396, w3390, w3389, w3388, w3387, 0.0 ("元素")) -> (w3400:dbl[])
                n2703 = call "多帧发送机制(EV05).vi"("can卡类型"=w3404, "设备索引号"=w3403, "CAN端口"=w3402, "命令"=w3398, "板号"=u8 0, "命令序号"=w3386, "输入数据"=w3400) -> ()  [unwired: 1 in, 12 out]
              }
              frame True {
                w3414 = 256.0 ("y")
                w3406 = u32 2 ("命令序号")
                w3418 = u8 192 ("命令")
                n2704 = local read "动作保持时间"() -> (w3415:dbl)
                n2705 = Quotient & Remainder(x=w3415, y=w3414) -> (x-y*floor(x/y)=w3407:dbl, floor(x/y)=w3411:dbl)
                n2706 = Quotient & Remainder(x=w3411, y=w3414) -> (x-y*floor(x/y)=w3408:dbl, floor(x/y)=w3412:dbl)
                n2707 = Quotient & Remainder(x=w3412, y=w3414) -> (x-y*floor(x/y)=w3409:dbl, floor(x/y)=w3413:dbl)
                n2708 = local read "设备索引号"() -> (w3423:u16)
                n2709 = local read "CAN卡类型"() -> (w3424:u32)
                n2710 = local read "CAN端口"() -> (w3422:u16)
                n2711 = Boolean To (0,1)(Boolean=w3419) -> (0, 1=w3416:i16)
                n2712 = Quotient & Remainder(x=w3413, y=w3414) -> (x-y*floor(x/y)=w3410:dbl)  [unwired: 1 out]
                n2713 = Build Array(i16 2 ("元素"), w3416, w3410, w3409, w3408, w3407, 0.0 ("元素")) -> (w3420:dbl[])
                n2714 = call "多帧发送机制(EV05).vi"("can卡类型"=w3424, "设备索引号"=w3423, "CAN端口"=w3422, "命令"=w3418, "板号"=u8 0, "命令序号"=w3406, "输入数据"=w3420) -> ()  [unwired: 1 in, 12 out]
              }
            }
            n2715 = local write "命令序号"(w3378) -> ()
            n2716 = local write "命令"(w3383) -> ()
            n2717 = local write "控制1"(TRUE ("控制1")) -> ()
            n2718 = local write "写?"(FALSE ("写?")) -> ()
            n2719 = local write "消除"(TRUE ("消除")) -> ()
            n2720 = global write "EV05全局变量1.vi" "流控帧 2"(TRUE ("流控帧 2")) -> ()
            n2721 = global write "EV05全局变量1.vi" "流控帧"(FALSE ("流控帧")) -> ()
          }
          frame #2 {
            n2722 = flat-sequence {
              tunnel: [w3426] -> w3425
              tunnel: w3425 -> [w3433]
              frame #0 {
                n2723 = while {
                  tunnel: [w3427] -> w3426
                  i -> [w3431]
                  stop <- w3428 stop-if-true
                  n2724 = local read "继电器超时处理"() -> (w3427:bool)
                  n2725 = Greater Or Equal?(x=w3431, y=20) -> (x >= y?=w3429:bool)
                  n2726 = Wait Until Next ms Multiple(millisecond multiple=u32 100 ("毫秒倍数")) -> ()  [unwired: 1 out]
                  n2727 = Or(x=w3427, y=w3429) -> (x .or. y?=w3428:bool)
                }
              }
              frame #1 {
                n2728 = case shown="假" w3433 {
                  frame False {
                    n2729 = local read "DO2"() -> (w3435:bool)
                    n2730 = Not(x=w3435) -> (.not. x?=w3434:bool)
                    n2731 = local write "DO2"(w3434) -> ()
                    n2732 = One Button Dialog(message="DO控制处理超时" ("消息"), button name ("OK")="是" ("按钮名称（“确定”）")) -> ()  [unwired: 1 out]
                  }
                  frame True {
                  }
                }
              }
            }
          }
        }
      }
      event "DO1 2": Value Change {
        n2733 = event-data() -> ("NewVal"=w3438:bool)  [unwired: 6 out]
        n2734 = stacked-sequence {
          tunnel: w3438 -> [_ w3452 _]
          frame #0 {
            w3441 = FALSE ("继电器超时处理")
            n2735 = local write "继电器超时处理"(w3441) -> ()
            n2736 = local write "正级继电器 11"(w3441) -> ()
            n2737 = local write "主从选择"(enum32{"主板", "从板"}."从板" ("主从选择")) -> ()
          }
          frame #1 {
            n2738 = case shown="假" w3452 {
              selector: w3452 -> [w3467 w3487]
              tunnel: [w3466 w3486] -> w3451
              tunnel: [w3465 w3485] -> w3445
              tunnel: [w3454 w3474] -> w3446
              frame True {
                w3462 = 256.0 ("y")
                w3454 = u32 2 ("命令序号")
                w3466 = u8 192 ("命令")
                n2739 = local read "动作保持时间"() -> (w3463:dbl)
                n2740 = Quotient & Remainder(x=w3463, y=w3462) -> (x-y*floor(x/y)=w3455:dbl, floor(x/y)=w3459:dbl)
                n2741 = Quotient & Remainder(x=w3459, y=w3462) -> (x-y*floor(x/y)=w3456:dbl, floor(x/y)=w3460:dbl)
                n2742 = Quotient & Remainder(x=w3460, y=w3462) -> (x-y*floor(x/y)=w3457:dbl, floor(x/y)=w3461:dbl)
                n2743 = Quotient & Remainder(x=w3461, y=w3462) -> (x-y*floor(x/y)=w3458:dbl)  [unwired: 1 out]
                n2744 = Boolean To (0,1)(Boolean=w3467) -> (0, 1=w3464:i16)
                n2745 = local read "设备索引号"() -> (w3471:u16)
                n2746 = local read "CAN卡类型"() -> (w3472:u32)
                n2747 = local read "从板板号"() -> (w3465:u8)
                n2748 = local read "CAN端口"() -> (w3470:u16)
                n2749 = Build Array(i16 3 ("元素"), w3464, w3458, w3457, w3456, w3455, 0.0 ("元素")) -> (w3469:dbl[])
                n2750 = call "多帧发送机制(EV05).vi"("can卡类型"=w3472, "设备索引号"=w3471, "CAN端口"=w3470, "命令"=w3466, "板号"=w3465, "命令序号"=w3454, "输入数据"=w3469) -> ()  [unwired: 1 in, 12 out]
              }
              frame False {
                w3482 = 256.0 ("y")
                w3474 = u32 2 ("命令序号")
                w3486 = u8 192 ("命令")
                n2751 = local read "动作保持时间"() -> (w3483:dbl)
                n2752 = Quotient & Remainder(x=w3483, y=w3482) -> (x-y*floor(x/y)=w3475:dbl, floor(x/y)=w3479:dbl)
                n2753 = Quotient & Remainder(x=w3479, y=w3482) -> (x-y*floor(x/y)=w3476:dbl, floor(x/y)=w3480:dbl)
                n2754 = Quotient & Remainder(x=w3480, y=w3482) -> (x-y*floor(x/y)=w3477:dbl, floor(x/y)=w3481:dbl)
                n2755 = Quotient & Remainder(x=w3481, y=w3482) -> (x-y*floor(x/y)=w3478:dbl)  [unwired: 1 out]
                n2756 = Boolean To (0,1)(Boolean=w3487) -> (0, 1=w3484:i16)
                n2757 = local read "设备索引号"() -> (w3491:u16)
                n2758 = local read "CAN卡类型"() -> (w3492:u32)
                n2759 = local read "从板板号"() -> (w3485:u8)
                n2760 = local read "CAN端口"() -> (w3490:u16)
                n2761 = Build Array(i16 1 ("元素"), w3484, w3478, w3477, w3476, w3475, 0.0 ("元素")) -> (w3489:dbl[])
                n2762 = call "多帧发送机制(EV05).vi"("can卡类型"=w3492, "设备索引号"=w3491, "CAN端口"=w3490, "命令"=w3486, "板号"=w3485, "命令序号"=w3474, "输入数据"=w3489) -> ()  [unwired: 1 in, 12 out]
              }
            }
            n2763 = local write "从板板号"(w3445) -> ()
            n2764 = local write "命令序号"(w3446) -> ()
            n2765 = local write "命令"(w3451) -> ()
            n2766 = local write "清BUFF"(FALSE ("清BUFF")) -> ()
            n2767 = local write "写?"(FALSE ("写?")) -> ()
            n2768 = local write "控制1"(TRUE ("控制1")) -> ()
            n2769 = global write "EV05全局变量1.vi" "流控帧"(FALSE ("流控帧")) -> ()
            n2770 = global write "EV05全局变量1.vi" "流控帧 2"(TRUE ("流控帧 2")) -> ()
            n2771 = local write "消除"(TRUE ("消除")) -> ()
          }
          frame #2 {
            n2772 = flat-sequence {
              tunnel: [w3494] -> w3493
              tunnel: w3493 -> [w3501]
              frame #0 {
                n2773 = while {
                  tunnel: [w3495] -> w3494
                  i -> [w3499]
                  stop <- w3496 stop-if-true
                  n2774 = local read "继电器超时处理"() -> (w3495:bool)
                  n2775 = Greater Or Equal?(x=w3499, y=20) -> (x >= y?=w3497:bool)
                  n2776 = Wait Until Next ms Multiple(millisecond multiple=u32 100 ("毫秒倍数")) -> ()  [unwired: 1 out]
                  n2777 = Or(x=w3495, y=w3497) -> (x .or. y?=w3496:bool)
                }
              }
              frame #1 {
                n2778 = case shown="假" w3501 {
                  frame False {
                    n2779 = local read "DO1 2"() -> (w3503:bool)
                    n2780 = Not(x=w3503) -> (.not. x?=w3502:bool)
                    n2781 = local write "DO1 2"(w3502) -> ()
                    n2782 = One Button Dialog(message="DO控制处理超时" ("消息"), button name ("OK")="是" ("按钮名称（“确定”）")) -> ()  [unwired: 1 out]
                  }
                  frame True {
                  }
                }
              }
            }
          }
        }
      }
      event "读取转换为写入": Value Change {
        n2783 = event-data() -> ("NewVal"=w3506:bool)  [unwired: 6 out]
        n2784 = case shown="真" w3506 {
          tunnel: w3510 -> [w3512 w3517]
          tunnel: [w3512 w3516] -> w3509
          tunnel: w3508 -> [w3511 w3515]
          tunnel: [w3511 w3514] -> w3507
          frame False {
          }
          frame True {
            n2785 = Enqueue Element(queue=w3517, element="读取转换为写入", error in (no error)=w3515) -> (queue out=w3516:refnum<queue>, error out=w3514:errorcluster)  [unwired: 2 out]
          }
        }
      }
      event "读取故障详细状态": Value Change {
        n2786 = event-data() -> ("NewVal"=w3522:bool)  [unwired: 5 out]
        n2787 = case shown="真" w3522 {
          tunnel: w3521 -> [w3524 w3537]
          tunnel: w3520 -> [w3523 w3536]
          tunnel: [w3524 w3535] -> w3519
          tunnel: [w3523 w3534] -> w3518
          frame False {
          }
          frame True {
            n2788 = disable-structure shown="启用" {
              disable-tunnel: [w3546 TRUE ("发送成功")] -> w3533
              frame Disabled {
                n2789 = local read "主从选择"() -> (w3538:enum32{"主板", "从板"})
                n2790 = case shown="\"主板\", 默认" w3538 {
                  tunnel: [0.0 ("FUNC") w3548] -> w3543
                  frame "主板", Default {
                  }
                  frame "从板" {
                    n2791 = local read "从板号"() -> (w3548:u8)
                  }
                }
                n2792 = local read "设备索引号"() -> (w3540:u16)
